vi "Strip Build Number.vi"(11 "Version String In":string) -> (3 "Version String":string)   [LabVIEW 2020, in "GCentral-API.lvlib"]
uses:
  GCentral-API.lvlib
  <vilib>/regexp/Match Regular Expression.xnode
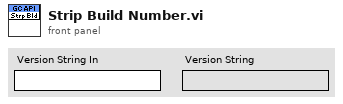
[diagram p1: front panel]
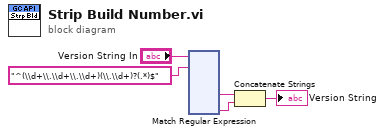
[diagram p0: block diagram]
diagram:
  n1 = xnode "Match Regular Expression"("input string"="Version String In", "regular expression"="^(\\d+\\.\\d+\\.\\d+)(\\.\\d+)?(.*)$") -> ("submatch 1"=w3:string, "submatch 3"=w2:string)  [unwired: 4 in, 6 out]
  n2 = Concatenate Strings(w3, w2) -> (→"Version String":string)
